vi "P Loop.vi"() -> ()   [LabVIEW 2016]
panel:
  out "Right Graph":dbl[](graph)
  out "Left Graph":dbl[](graph)
  in  "Scaling Factor":dbl
  out "Right Power":dbl
  in  "Gyro Angle":dbl
  out "Left Motor Power":dbl
  in  "stop":bool
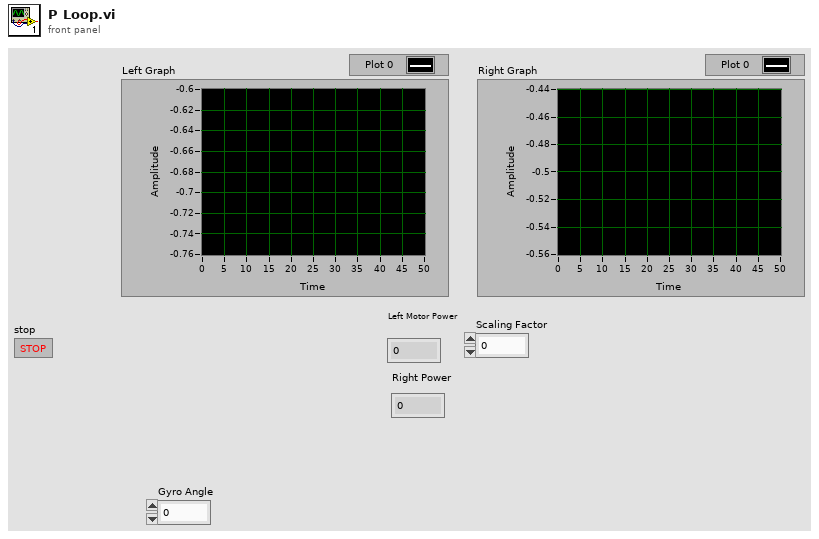
[diagram p1: front panel]
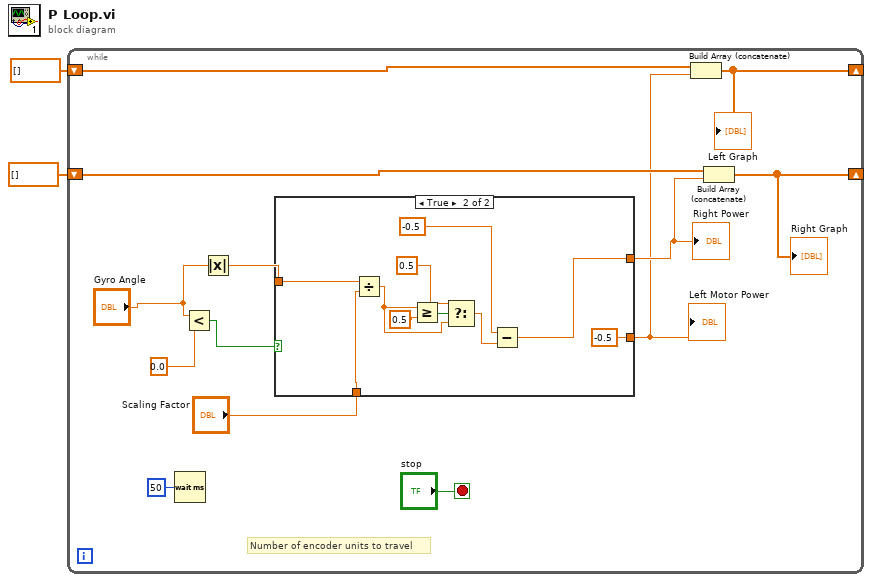
[diagram p0: block diagram]
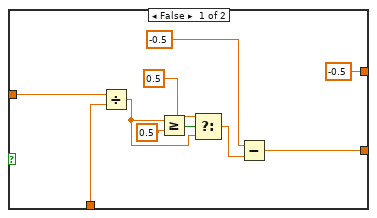
[diagram p2: hidden frame]
diagram:
  n1 = while {
    shift-right: [w7] -> _
    shift-left: dbl[] [] -> [w5]
    shift-right: [w4] -> _
    shift-left: dbl[] [] -> [w8]
    stop <- "stop" stop-if-true
    # "Number of encoder units to travel"
    n2 = Wait (ms)(milliseconds to wait=u32 50) -> ()  [unwired: 1 out]
    n3 = Less?(x="Gyro Angle", y=0.0) -> (x < y?=w12:bool)
    n4 = Absolute Value(x="Gyro Angle") -> (abs(x)=w11:dbl)
    n5 = case shown="True" w12 {
      tunnel: w11 -> [w19 w29]
      tunnel: [w18 -0.5] -> w6
      tunnel: [-0.5 w28] -> w9
      tunnel: "Scaling Factor" -> [w16 w26]
      frame False {
        n6 = Divide(x=w19, y=w16) -> (x/y=w20:dbl)
        n7 = Greater Or Equal?(x=w20, y=0.5) -> (x >= y?=w24:bool)
        n8 = Select(t=0.5, s=w24, f=w20) -> (s? t:f=w21:dbl)
        n9 = Subtract(x=-0.5 ("y"), y=w21) -> (x-y=w18:dbl)
      }
      frame True {
        n10 = Divide(x=w29, y=w26) -> (x/y=w30:dbl)
        n11 = Greater Or Equal?(x=w30, y=0.5) -> (x >= y?=w34:bool)
        n12 = Select(t=0.5, s=w34, f=w30) -> (s? t:f=w31:dbl)
        n13 = Subtract(x=-0.5 ("y"), y=w31) -> (x-y=w28:dbl)
      }
    }
    "Left Motor Power" <- w6
    "Right Power" <- w9
    n14 = Build Array (concatenate)(w5, w6) -> (w7:dbl[])
    "Left Graph" <- w7
    n15 = Build Array (concatenate)(w8, w9) -> (w4:dbl[])
    "Right Graph" <- w4
  }
